vi "Read Measurement (Ripple Power Analysis).vi"(0 "VISA resource name":refnum<visa-resource-name>, 11 "error in (no error)":errorcluster) -> (4 "VISA resource name out":refnum<visa-resource-name>, 6 "Ripple Measurement":dbl, 15 "error out":errorcluster)   [LabVIEW 2015, in "Agilent 2000 3000 X-Series.lvlib"]
doc: "Returns the measurement of a ripple power analysis.\n\n<B>Note(s):</B>\nUse <B>Configure Power Analysis (Ripple).vi</B> to apply a power analysis."
uses:
  <instrlib>/Agilent 2000 3000 X-Series/Agilent 2000 3000 X-Series.lvlib
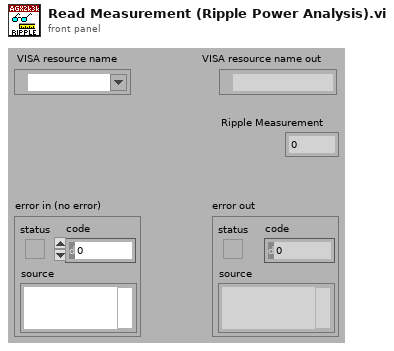
[diagram p1: front panel]
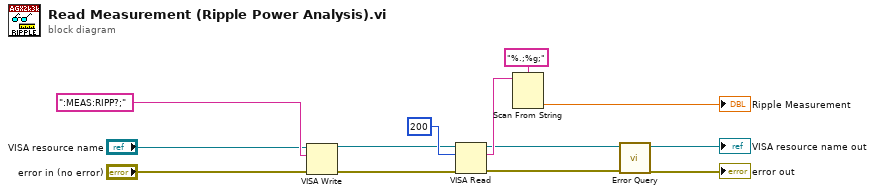
[diagram p0: block diagram]
diagram:
  n1 = VISA Write(VISA resource name="VISA resource name", write buffer=":MEAS:RIPP?;", error in (no error)="error in (no error)") -> (VISA resource name out=w6:refnum<visa-resource-name>, error out=w5:errorcluster)  [unwired: 1 out]
  n2 = VISA Read(VISA resource name=w6, byte count=u32 200, error in (no error)=w5) -> (VISA resource name out=w4:refnum<visa-resource-name>, read buffer=w7:string, error out=w3:errorcluster)  [unwired: 1 out]
  n3 = Scan From String(format string="%.;%g;", input string=w7) -> (output 1=→"Ripple Measurement":dbl)  [unwired: 2 in, 4 out]
  n4 = call <instrlib>:"Error Query.vi"("error in (no error)"=w3, "VISA resource name"=w4) -> ("error out"=→"error out":errorcluster, "VISA resource name out"=→"VISA resource name out":refnum<visa-resource-name>)  [unwired: 8 out]
